vi "Write--move.vi"(8 "error in (no error)":errorcluster, 10 "Comando":T1 {"Step style motor 2" items=["Medio paso", "Paso completo"]; "Step style motor 1" items=["Medio paso", "Paso completo"]; "Direction motor 2" items=["", "Forward", "Backward"]; "Direction motor 1" items=["", "Forward", "Backward"]; "Action" items=["Initialize", "Move"]}, 11 "VISA resource name":refnum<visa-resource-name>) -> (0 "error out":errorcluster, 2 "Comando(string)":string, 3 "VISA resource name out":refnum<visa-resource-name>)   [LabVIEW 2020, in "Control de MaP.lvlib"]
doc: "convierte la selección de comando a cadena y lo envía al puerto seleccionado"
uses:
  Control de MaP.lvlib
  Controls/Move motor parameters--cluster.ctl
  Controls/Motor direction.ctl
  Controls/Step style.ctl
  <vilib>/Instr/_visa.llb/VISA Flush IO Buffer Mask.ctl
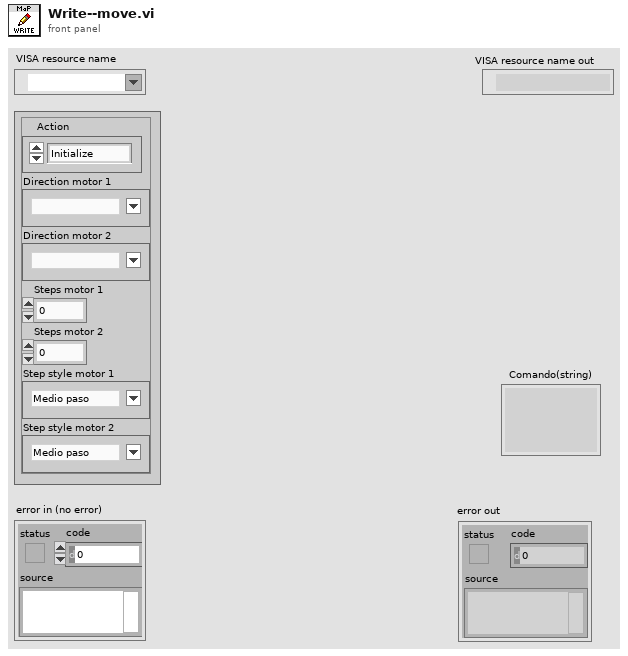
[diagram p1: front panel]
types:
  T1 = typedef "Control de MaP.lvlib/Move motor parameters--cluster.ctl" = cluster{"Action":u8, "Direction motor 1":T2, "Direction motor 2":T2, "Steps motor 1":u16, "Steps motor 2":u16, "Step style motor 1":T3, "Step style motor 2":T3}
  T2 = typedef "Control de MaP.lvlib/Motor direction.ctl" = u8
  T3 = typedef "Control de MaP.lvlib/Step style.ctl" = u8
  T4 = typedef "VISA Flush IO Buffer Mask.ctl" = u16
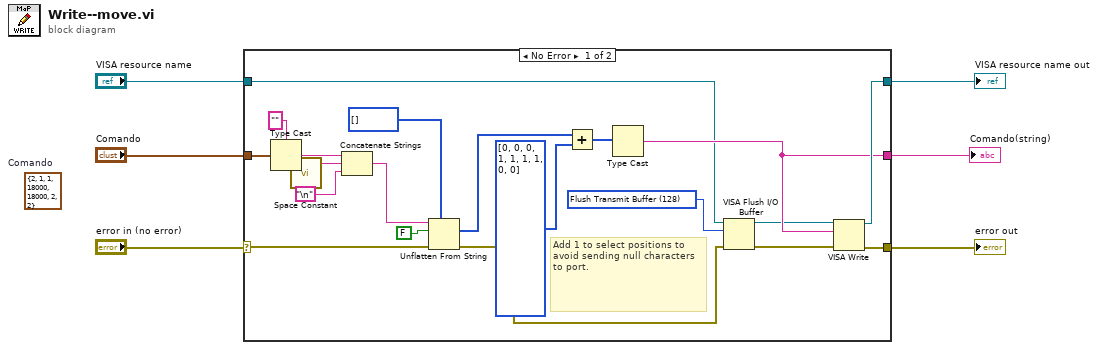
[diagram p0: block diagram]
diagram:
  (unwired) T1 {"Action"=2, "Direction motor 1"=1, "Direction motor 2"=1, "Steps motor 1"=18000, "Steps motor 2"=18000, "Step style motor 1"=2, "Step style motor 2"=2}  # Comando
  n1 = case shown="No Error" "error in (no error)" {
    selector: "error in (no error)" -> [w8 w28]
    tunnel: "VISA resource name" -> [w14 w27]
    tunnel: [w26 w27] -> w5
    tunnel: [w25 w28] -> w3
    tunnel: "Comando" -> [w24 _]
    tunnel: [w17 _] -> w1
    frame No Error {
      w16 = T4 128 items=["Flush Receive Buffer"=16, "Write Transmit Buffer to Device"=32, "Flush Receive Buffer (No I/O)"=64, "Flush Transmit Buffer"=128] ("Mask")
      # "Add 1 to select positions to avoid sending null characters to port."
      n2 = Type Cast(type="", x=w24) -> (*(type *) &x=w10:string)
      n3 = call <vilib>:"Space Constant.vi"() -> ("String"=w12:string)
      n4 = Concatenate Strings(w10, w12, "\n") -> (w9:string)
      n5 = Unflatten From String(type=u8[] [], binary string=w9, data includes array or string size? (T)=FALSE, error in (no error)=w8) -> (value=w20:u8[], error out=w7:errorcluster)  [unwired: 1 in, 1 out]
      n6 = Add(x=w20, y=u8[] [0, 0, 0, 1, 1, 1, 1, 0, 0]) -> (x+y=w18:u8[])
      n7 = Type Cast(x=w18) -> (*(type *) &x=w17:string)  [unwired: 1 in]
      n8 = VISA Flush I/O Buffer(VISA resource name=w14, mask (16)=w16, error in (no error)=w7) -> (VISA resource name out=w13:refnum<visa-resource-name>, error out=w15:errorcluster)
      n9 = VISA Write(VISA resource name=w13, write buffer=w17, error in (no error)=w15) -> (VISA resource name out=w26:refnum<visa-resource-name>, error out=w25:errorcluster)  [unwired: 1 out]
    }
    frame Error {
    }
  }
  "VISA resource name out" <- w5
  "error out" <- w3
  "Comando(string)" <- w1
